vi "DynamicMotionMagicTorqueCurrentFOC SetControl.vi"(0 "DeviceReference":T1, 1 "StopSendingOtherRequests":bool=TRUE, 2 "Position":dbl, 3 "Velocity":dbl, 4 "Acceleration":dbl, 5 "Jerk":dbl, 6 "FeedForward":dbl, 7 "error in":errorcluster, 8 "Slot":i32, 9 "OverrideCoastDurNeutral":bool, 10 "LimitForwardMotion":bool, 11 "LimitReverseMotion":bool, 18 "Update Frequency (Hz)":dbl=100.0) -> (20 "DeviceReference Out":T1, 27 "error out":errorcluster)   [LabVIEW 2023]
doc: "Requests Motion Magic® to target a final position using a motion profile. This dynamic request allows runtime changes to Cruise Velocity, Acceleration, and Jerk. Users can optionally provide a torque current feedforward. This control requires use of a CANivore.\nMotion Magic® produces a motion profile in real-time while attempting to honor the specified Cruise Velocity, Acceleration, and Jerk value. This control mode does not use the Expo_kV or Expo_kA configs. Target position can be changed on-the-fly and Motion Magic® will do its best to adjust the profile. This control mode is based on torque current, so relevant closed-loop gains will use Amperes for the numerator."
uses:
  <vilib>/Rock Robotics/WPI/ThirdParty/Phoenix6/DeviceReference.ctl
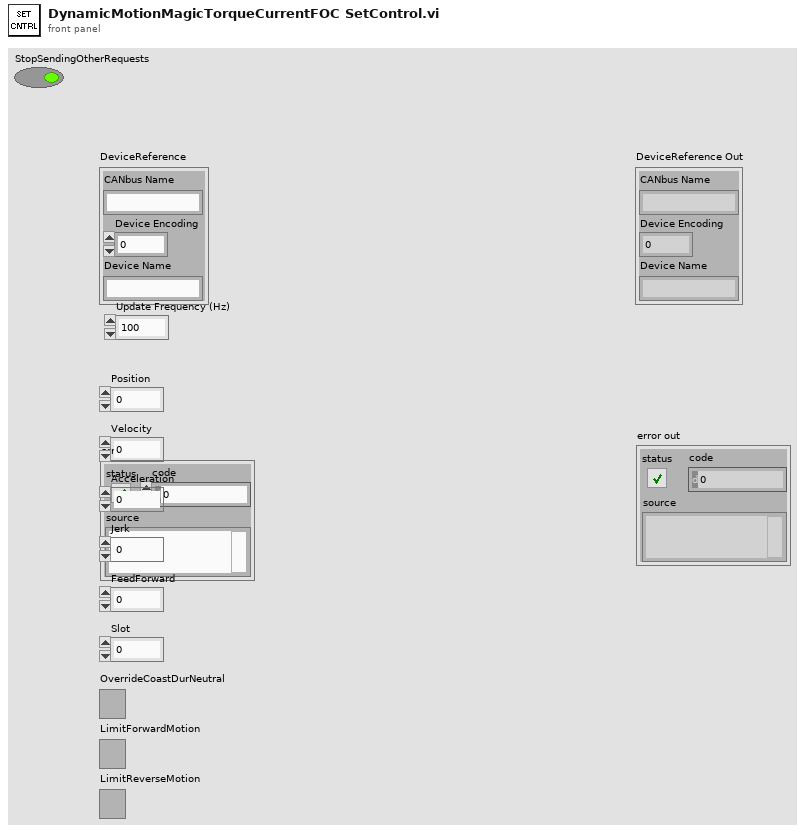
[diagram p1: front panel]
types:
  T1 = typedef "DeviceReference.ctl" = cluster{"CANbus Name":string, "Device Encoding":u32, "Device Name":string}
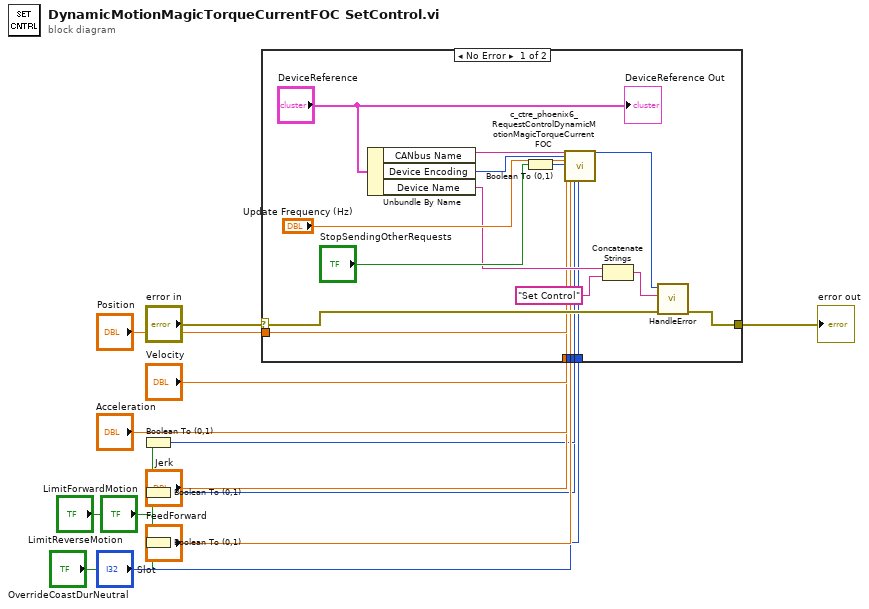
[diagram p0: block diagram]
diagram:
  n1 = Boolean To (0,1)(Boolean="OverrideCoastDurNeutral") -> (0, 1=w5:i16)
  n2 = Boolean To (0,1)(Boolean="LimitForwardMotion") -> (0, 1=w3:i16)
  n3 = Boolean To (0,1)(Boolean="LimitReverseMotion") -> (0, 1=w1:i16)
  n4 = case shown="No Error" "error in" {
    selector: "error in" -> [w28 w36]
    tunnel: [w27 w36] -> w13
    tunnel: "Position" -> [w23 _]
    tunnel: "Velocity" -> [w22 _]
    tunnel: "Acceleration" -> [w21 _]
    tunnel: "Jerk" -> [w20 _]
    tunnel: "FeedForward" -> [w19 _]
    tunnel: "Slot" -> [w18 _]
    tunnel: w5 -> [w17 _]
    tunnel: w3 -> [w16 _]
    tunnel: w1 -> [w15 _]
    frame No Error {
      n5 = Unbundle By Name("DeviceReference") -> ("CANbus Name"=w34:string, "Device Encoding"=w33:u32, "Device Name"=w26:string)
      n6 = Boolean To (0,1)(Boolean="StopSendingOtherRequests") -> (0, 1=w30:i16)
      n7 = call <vilib>:"c_ctre_phoenix6_RequestControlDynamicMotionMagicTorqueCurrentFOC.vi"("String 2"=w34, "Numeric 2"=w33, "Numeric 3"="Update Frequency (Hz)", "Numeric 4"=w30, "Numeric 5"=w23, "Numeric 6"=w22, "Numeric 7"=w21, "Numeric 8"=w20, "Numeric 9"=w19, "Numeric 10"=w18, "Numeric 11"=w17, "Numeric 12"=w16, "Numeric 13"=w15) -> ("Numeric"=w29:i32)  [unwired: 13 in, 1 out]
      n8 = Concatenate Strings(w26, "Set Control" ("origin")) -> (w24:string)
      n9 = call "HandleError.vi"("error in"=w28, "origin"=w24, "Status"=w29) -> ("error out"=w27:errorcluster)  [unwired: 8 in]
      "DeviceReference Out" <- "DeviceReference"
    }
    frame Error {
    }
  }
  "error out" <- w13
